vi "Read COM Port.vi"(8 "error in (no error)":errorcluster, 11 "AirMar in":refnum<class "AirMar.lvclass">) -> (0 "error out":errorcluster, 2 "COM Port":refnum<visa-resource-name>, 3 "AirMar out":refnum<class "AirMar.lvclass">)   [LabVIEW 2017, in "Sensors.lvlib" / "AirMar.lvclass"]
uses:
  AirMar.lvclass
  AirMar.lvclass/AirMar.ctl
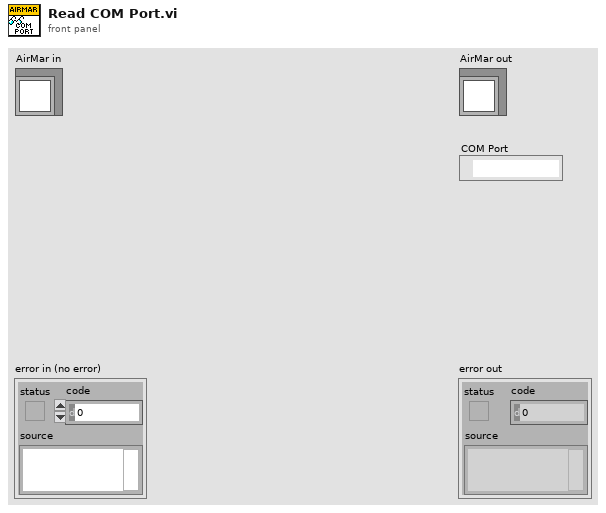
[diagram p1: front panel]
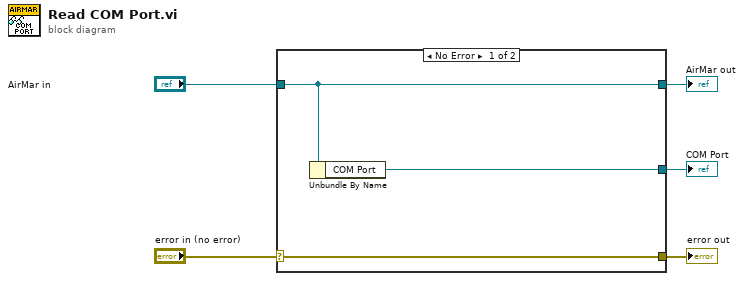
[diagram p0: block diagram]
diagram:
  n1 = case shown="No Error" "error in (no error)" {
    selector: "error in (no error)" -> [w8 w9]
    tunnel: [w8 w9] -> w4
    tunnel: [w7 w10] -> w2
    tunnel: "AirMar in" -> [w7 w10]
    tunnel: [w6 _] -> w1
    frame No Error {
      n2 = Unbundle By Name(w7) -> ("COM Port"=w6:refnum<visa-resource-name>)
    }
    frame Error {
    }
  }
  "error out" <- w4
  "AirMar out" <- w2
  "COM Port" <- w1
